vi "Move.vi"(7 "Oriel (custom drivers) in":T1, 8 "error in (no error)":errorcluster, 11 "Wavelength":dbl) -> (0 "error out":errorcluster, 1 "Wavelength Set":bool=TRUE, 5 "Oriel (custom drivers) out":T1)   [LabVIEW 2017, in "Monochromator.lvlib" / "Oriel (custom drivers).lvlib"]
uses:
  Oriel (custom drivers).lvlib
  Controls/Params.ctl
  C:/Project Work/icl-optical-software-rewrite/Optical Software Code Simplified/Modules/Monochromator/Cornerstone.dll
  Cornerstone.dll
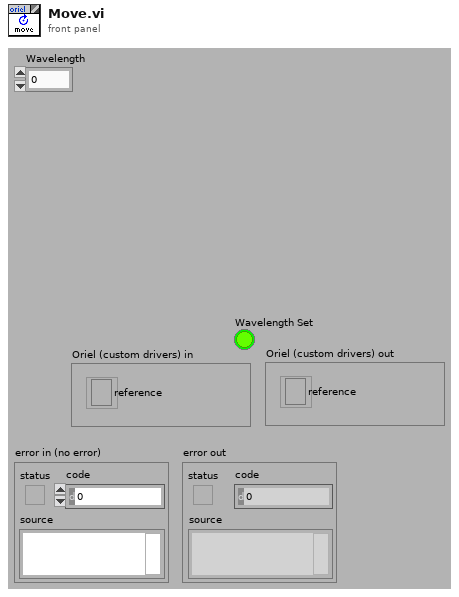
[diagram p1: front panel]
types:
  T1 = typedef "Monochromator.lvlib/Oriel (custom drivers).lvlib/Params.ctl" = cluster{"reference":refnum<k24>}
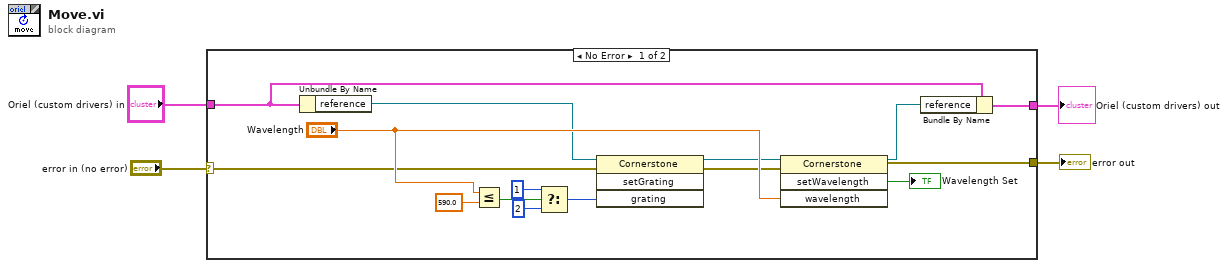
[diagram p0: block diagram]
diagram:
  n1 = case shown="No Error" "error in (no error)" {
    selector: "error in (no error)" -> [w10 w21]
    tunnel: [w19 w21] -> w3
    tunnel: [w17 w20] -> w2
    tunnel: "Oriel (custom drivers) in" -> [w15 w20]
    frame No Error {
      n2 = Unbundle By Name(w15) -> ("reference"=w12:refnum<k24>)
      n3 = Less Or Equal?(x="Wavelength", y=590.0) -> (x <= y?=w7:bool)
      n4 = Select(t=1, s=w7, f=2) -> (s? t:f=w9:i32)
      n5 = invoke class="Cornerstone" method="setGrating"(reference=w12, error in=w10, "grating"=w9) -> (reference out=w11:refnum<k24>, error out=w13:errorcluster)  [unwired: 1 in, 2 out]
      n6 = invoke class="Cornerstone" method="setWavelength"(reference=w11, error in=w13, "wavelength"="Wavelength") -> (reference out=w16:refnum<k24>, error out=w19:errorcluster, "setWavelength"=→"Wavelength Set":bool)  [unwired: 1 in, 1 out]
      n7 = Bundle By Name(cluster=w15, "reference"=w16) -> (w17:T1)
    }
    frame Error {
    }
  }
  "error out" <- w3
  "Oriel (custom drivers) out" <- w2
